vi "Configure Percent Math Calculation.vi"(8 "error in (no error)":errorcluster, 9 "Use Input Signal as Target Value (F: Disable)":bool, 10 "Target Value (1)":dbl=1.0, 11 "VISA resource name":refnum<visa-resource-name>) -> (0 "error out":errorcluster, 3 "VISA resource name out":refnum<visa-resource-name>)   [LabVIEW 2011, in "Keithley 2182.lvlib"]
doc: "Configures the percent math calculation.\n\nThis math function determines percent deviation from a specified reference value. The percent calculation is performed as follows:\n\n<B> Input - Reference\nPercent = ______________________________ * 100%\n Reference\n </B>where:\n <B>Input</B> is the normal display reading\n <B>Reference</B> is the user entered constant\n <B>Percent</B> is the displayed result"
uses:
  Keithley 2182.lvlib
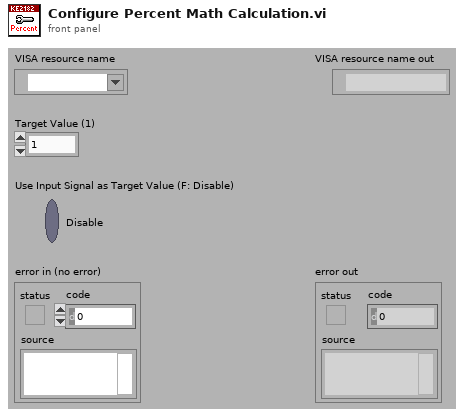
[diagram p1: front panel]
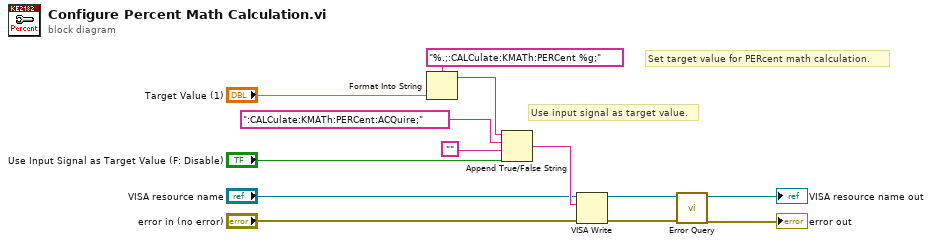
[diagram p0: block diagram]
diagram:
  # "Use input signal as target value."
  # "Set target value for PERcent math calculation."
  n1 = Format Into String(format string="%.;:CALCulate:KMATh:PERCent %g;", "Target Value (1)") -> (resulting string=w11:string)  [unwired: 2 in, 1 out]
  n2 = Append True/False String(1:"Use Input Signal as Target Value (F: Disable)", 2:"", 3:":CALCulate:KMATh:PERCent:ACQuire;", 4:w11) -> (0:w8:string)
  n3 = VISA Write(VISA resource name="VISA resource name", write buffer=w8, error in (no error)="error in (no error)") -> (VISA resource name out=w5:refnum<visa-resource-name>, error out=w4:errorcluster)  [unwired: 1 out]
  n4 = call "Error Query.vi"("error in (no error)"=w4, "VISA resource name"=w5) -> ("error out"=→"error out":errorcluster, "VISA resource name out"=→"VISA resource name out":refnum<visa-resource-name>)  [unwired: 6 in, 2 out]
